vi "Demo Ring and Enum.vi"(8 "error in (no error)":errorcluster) -> (0 "error out":errorcluster)   [LabVIEW 2011]
uses:
  VIremote.llb/VIremoteEvent.ctl
  VIremote.llb/VIremoteFunction.ctl
  VIremote.llb/VIremoteStatus.ctl
panel:
  in  "Ring Grouped 3":sgl(ring)=1.0 caption="Picker" items=["-Header 1", "First Item", "Second Item (with detail text)", "Grey Item (disabled) ", "-Header 2", "something", "somethingelse", "-Header 3", "Some Item", "Some other Item", "/Footer"]
  in  "VIremoteEvent":T1=enum."Connection Closed"
  in  "Ring Grouped 2":sgl(ring)=1.0 caption="Menu Ring Plain" items=["-Header 1", "First Item", "Second Item (with detail text)", "Grey Item (disabled) ", "-Header 2", "something", "somethingelse", "-Header 3", "Some Item", "Some other Item", "/Footer"]
  in  "Enum Grouped":enum32{"First", "Second", "Third"}(ring) caption="Enum"
  in  "Text Ring Grouped":u16(ring) items=["Number one", "Number two", "Number three", "-", "Number 44", "Number 45", "Number 46"]
  in  "Text Ring":u16(ring)=1 items=["-First Header", "Number one", "Number two", "Number three", "-Second Header", "Number 44", "Number 45", "Number 46"]
  in  "Enum":T2(ring)
  in  "Ring Grouped":sgl(ring)=1.0 caption="Grouped" items=["-Header 1", "First Item", "Second Item (with detail text)", "Grey Item (disabled) ", "-Header 2", "something", "somethingelse", "-Header 3", "Some Item", "Some other Item", "/Footer"]
  # "Tap this to display a native iOS table view. Create sections by using the '-' character. If you want a header text you can enter it after the '-' character and disable the item. Footers can be entered in the same way after a '/' character.\nThe text in the title bar is taken from the Caption.\nIf you include the string \"Style=Grouped\" or \"Style=Picker\" after \"VIREMOTEPROPERTIES\" in the description of the control it will be displayed like the two below.\n\n(See Demo BG Notification and Status.vi, Demo File Dialog.vi and All_Demos.vi for other examples of using menu rings)"
  # "Disabled items will not show up in a picker"
  # "Text rings work the same as menu rings except they have optional Increment/Decrement buttons that can't be used by VIremote."
  # "Section splitters in enums must use the -Headertext syntax as every value has to be unique ('-' could be used once)."
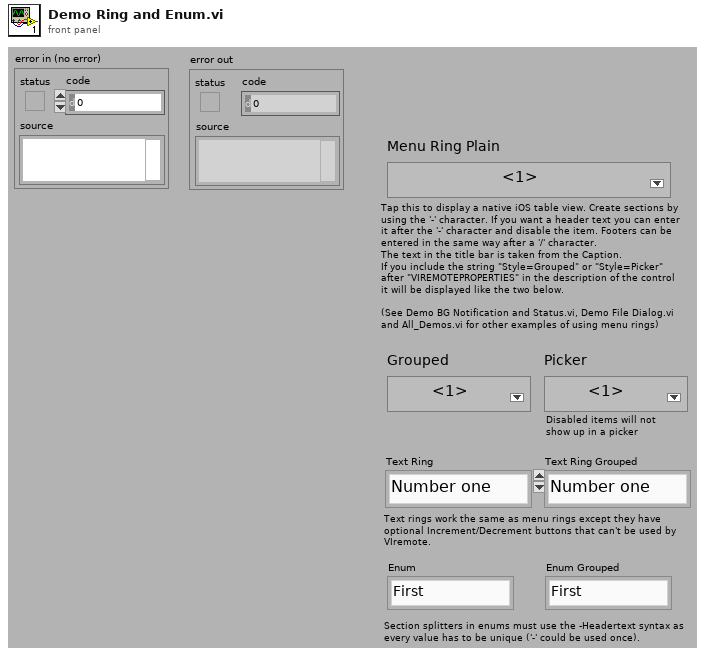
[diagram p1: front panel]
types:
  T1 = typedef "VIremoteEvent.ctl" = enum16{"No Event", "Connection Closed", "Navigate Back", "Enter Background", "Enter Foreground", "Portrait", "Portrait Upside Down", "Landscape Left", "Landscape Right"}
  T2 = enum32{"First", "Second", "Third", "-Fourth is a Header", "Fifth", "Sixth"}
  T3 = typedef "VIremoteStatus.ctl" = enum16{"Connected BOOL", "Number of connections DBL", "VIremoteController ver.", "VIremote ver. DBL", "Screen width DBL", "Screen height DBL", "Current navigation bar height DBL", "Current UI orientation", "Background supported BOOL", "Background state BOOL", "Device UI idiom (0=phone,1=iPad) DBL", "Device name", "Device unique id", "Device system ver.", "Device model", "Device HW model"}
  T4 = typedef "VIremoteFunction.ctl" = enum16{"Do nothing", "Stop controller", "Close this connection", "Show info panel", "Set VI to control", "Set Accelerometer freq (Hz)", "Show Alert message", "Start Sound Input", "Stop Sound Input", "Set Volume (0-100)", "Set sound output Speaker", "Set sound output Receiver", "Play Sound", "Repeat Sound", "Stop Sound", "Pause Sound", "Resume Sound", "Set panel width of caller (320 or 480)", "Set Panel Size to Portrait", "Set Panel Size to Landscape", "Set Panel Size as Current Orientation", "Allow all UI Orientations", "Send user notification", "Disable Scrolling", "Normal Scrolling", "Page Scrolling", "Set Scroll Offset", "Page Indicator Position"}
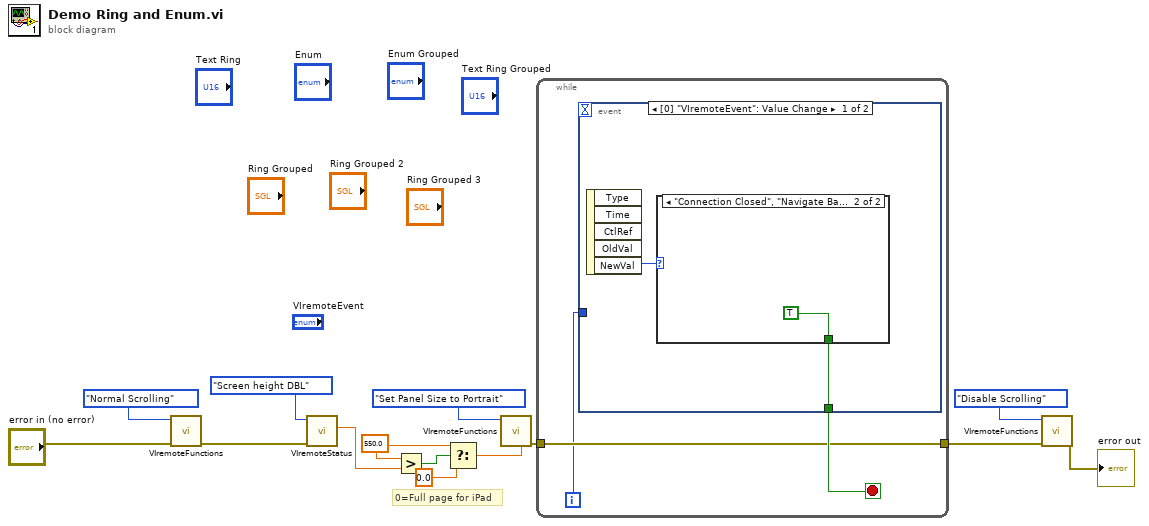
[diagram p0: block diagram]
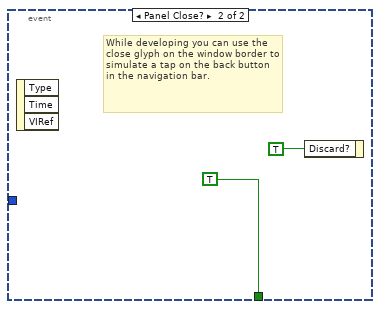
[diagram p3: hidden frame]
diagram:
  w3 = 550.0 ("Value in Y")
  # "0=Full page for iPad"
  n1 = call "VIremoteFunctions.vi"("error in (no error)"="error in (no error)", "Function"=VIremoteFunction."Normal Scrolling") -> ("error out"=w6:errorcluster)  [unwired: 4 in, 5 out]
  n2 = call "VIremoteStatus.vi"("error in (no error)"=w6, "Status item"=VIremoteStatus."Screen height DBL") -> ("DBL"=w5:dbl)  [unwired: 1 in, 8 out]
  n3 = Greater?(x=w3, y=w5) -> (0:w4:bool)
  n4 = Select(t=w3, s=w4, f=0.0) -> (s? t:f=w1:dbl)
  n5 = call "VIremoteFunctions.vi"("Value in Y"=w1, "Function"=VIremoteFunction."Set Panel Size to Portrait") -> ("error out"=w9:errorcluster)  [unwired: 4 in, 5 out]
  n6 = while {
    tunnel: w9 -> [w16]
    tunnel: [w16] -> w8
    i -> [w15]
    stop <- w17 stop-if-true
    n7 = event shown="[0] \"VIremoteEvent\": Value Change" {
      selector: _ -> [_ _]
      dyn-events: _ -> [_ _]
      timeout: _ -> [_ _]
      tunnel: [w18 TRUE ("Discard?")] -> w17
      tunnel: w15 -> [_ _]
      event Value Change {
        n8 = event-data() -> ("NewVal"=w19:T1)  [unwired: 5 out]
        n9 = case shown="\"Connection Closed\", \"Navigate Back\"" w19 {
          tunnel: [_ TRUE] -> w18
          frame "No Event", Default {
          }
          frame "Connection Closed", "Navigate Back" {
          }
        }
      }
      event Panel Close? {
        # "While developing you can use the close glyph on the window border to simulate a tap on the back button in the navigation bar."
        n10 = event-data() -> ()  [unwired: 4 out]
        n11 = event-data("Discard?"=TRUE) -> ()  [unwired: 1 in, 1 out]
      }
    }
  }
  n12 = call "VIremoteFunctions.vi"("error in (no error)"=w8, "Function"=VIremoteFunction."Disable Scrolling") -> ("error out"=→"error out":errorcluster)  [unwired: 4 in, 5 out]
